vi "GVmotor_move_DIFL.vi"(8 "error in":errorcluster, 9 "relative_step":i32, 10 "wait_ms":u32=100, 11 "VISA in":refnum<visa-resource-name>) -> (0 "error out":errorcluster, 3 "VISA out":refnum<visa-resource-name>)   [LabVIEW 2019]
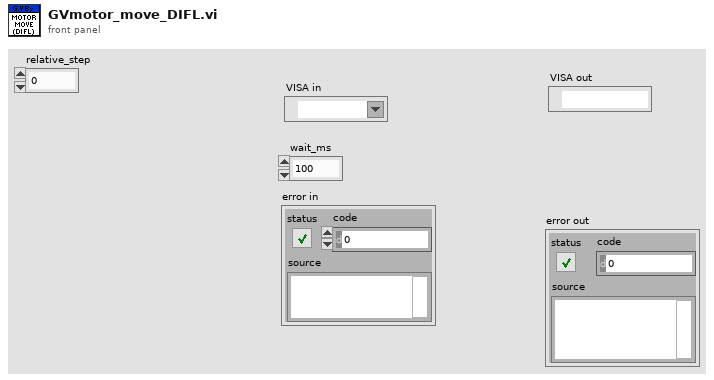
[diagram p1: front panel]
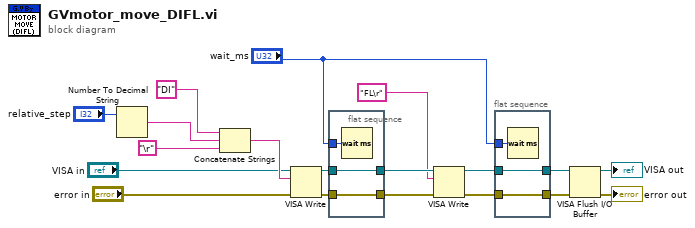
[diagram p0: block diagram]
diagram:
  n1 = Number To Decimal String(number="relative_step") -> (decimal integer string=w13:string)  [unwired: 1 in]
  n2 = Concatenate Strings("DI" ("string"), w13, "\r") -> (w19:string)
  n3 = VISA Write(VISA resource name="VISA in", write buffer=w19, error in (no error)="error in") -> (VISA resource name out=w15:refnum<visa-resource-name>, error out=w16:errorcluster)  [unwired: 1 out]
  n4 = flat-sequence {
    tunnel: [w22] -> w6
    tunnel: w16 -> [w22]
    tunnel: [w21] -> w7
    tunnel: w15 -> [w21]
    tunnel: "wait_ms" -> [w20]
    frame #0 {
      n5 = Wait (ms)(milliseconds to wait=w20) -> ()  [unwired: 1 out]
    }
  }
  n6 = VISA Write(VISA resource name=w7, write buffer="FL\r" ("string"), error in (no error)=w6) -> (VISA resource name out=w5:refnum<visa-resource-name>, error out=w4:errorcluster)  [unwired: 1 out]
  n7 = flat-sequence {
    tunnel: [w25] -> w3
    tunnel: w4 -> [w25]
    tunnel: [w24] -> w8
    tunnel: w5 -> [w24]
    tunnel: [w23] -> _
    tunnel: "wait_ms" -> [w23]
    frame #0 {
      n8 = Wait (ms)(milliseconds to wait=w23) -> ()  [unwired: 1 out]
    }
  }
  n9 = VISA Flush I/O Buffer(VISA resource name=w8, error in (no error)=w3) -> (VISA resource name out=→"VISA out":refnum<visa-resource-name>, error out=→"error out":errorcluster)  [unwired: 1 in]
